vi "外部交互全局.vi"() -> ()   [LabVIEW 2022 SP3, in "超标留样集成.lvlib"]
panel:
  out "采配水流程":T1(ring)=enum."结束"
  in  "当前瓶号":u16
  out "超标留样信号":bool
  in  "CODCr超标浓度":dbl
  in  "CODMn超标浓度":dbl
  in  "总氮超标浓度":dbl
  in  "总磷超标浓度":dbl
  in  "氨氮超标浓度":dbl
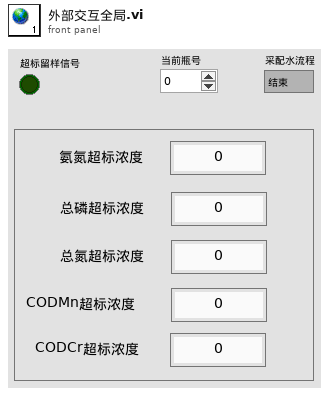
[diagram p1: front panel]
types:
  T1 = enum16{"空闲", "润洗", "采样", "沉淀", "配水", "反冲洗", "储水", "结束"}
diagram:
